vi "Edit_Batch.vi"(6 "error in (no error) 5":errorcluster, 7 "Batch Data 3":T1, 8 "Primery key names":string[](array[string]), 9 "Module Number  3":dbl=1.0, 10 "Batch data":string[](array[string]), 11 "Primery key last values":string[](array[string])) -> (0 "error out":errorcluster, 3 "Sucess ?":bool)   [LabVIEW 2015, in "Copy of Untitled Library 1.lvlib"]
uses:
  Copy of Untitled Library 1.lvlib
  Controls/Caller Queue Control .ctl
  Controls/Control 1.ctl
  Controls/Enum Constant.ctl
  <userlib>/origin_lib_main/db_interface/DB Operations Enum.ctl
  <userlib>/origin_lib_main/db_interface/DB Interface.lvlib
panel:
  in  "Cluster":T2
  out "concatenated string":string
  out "format string 2":string
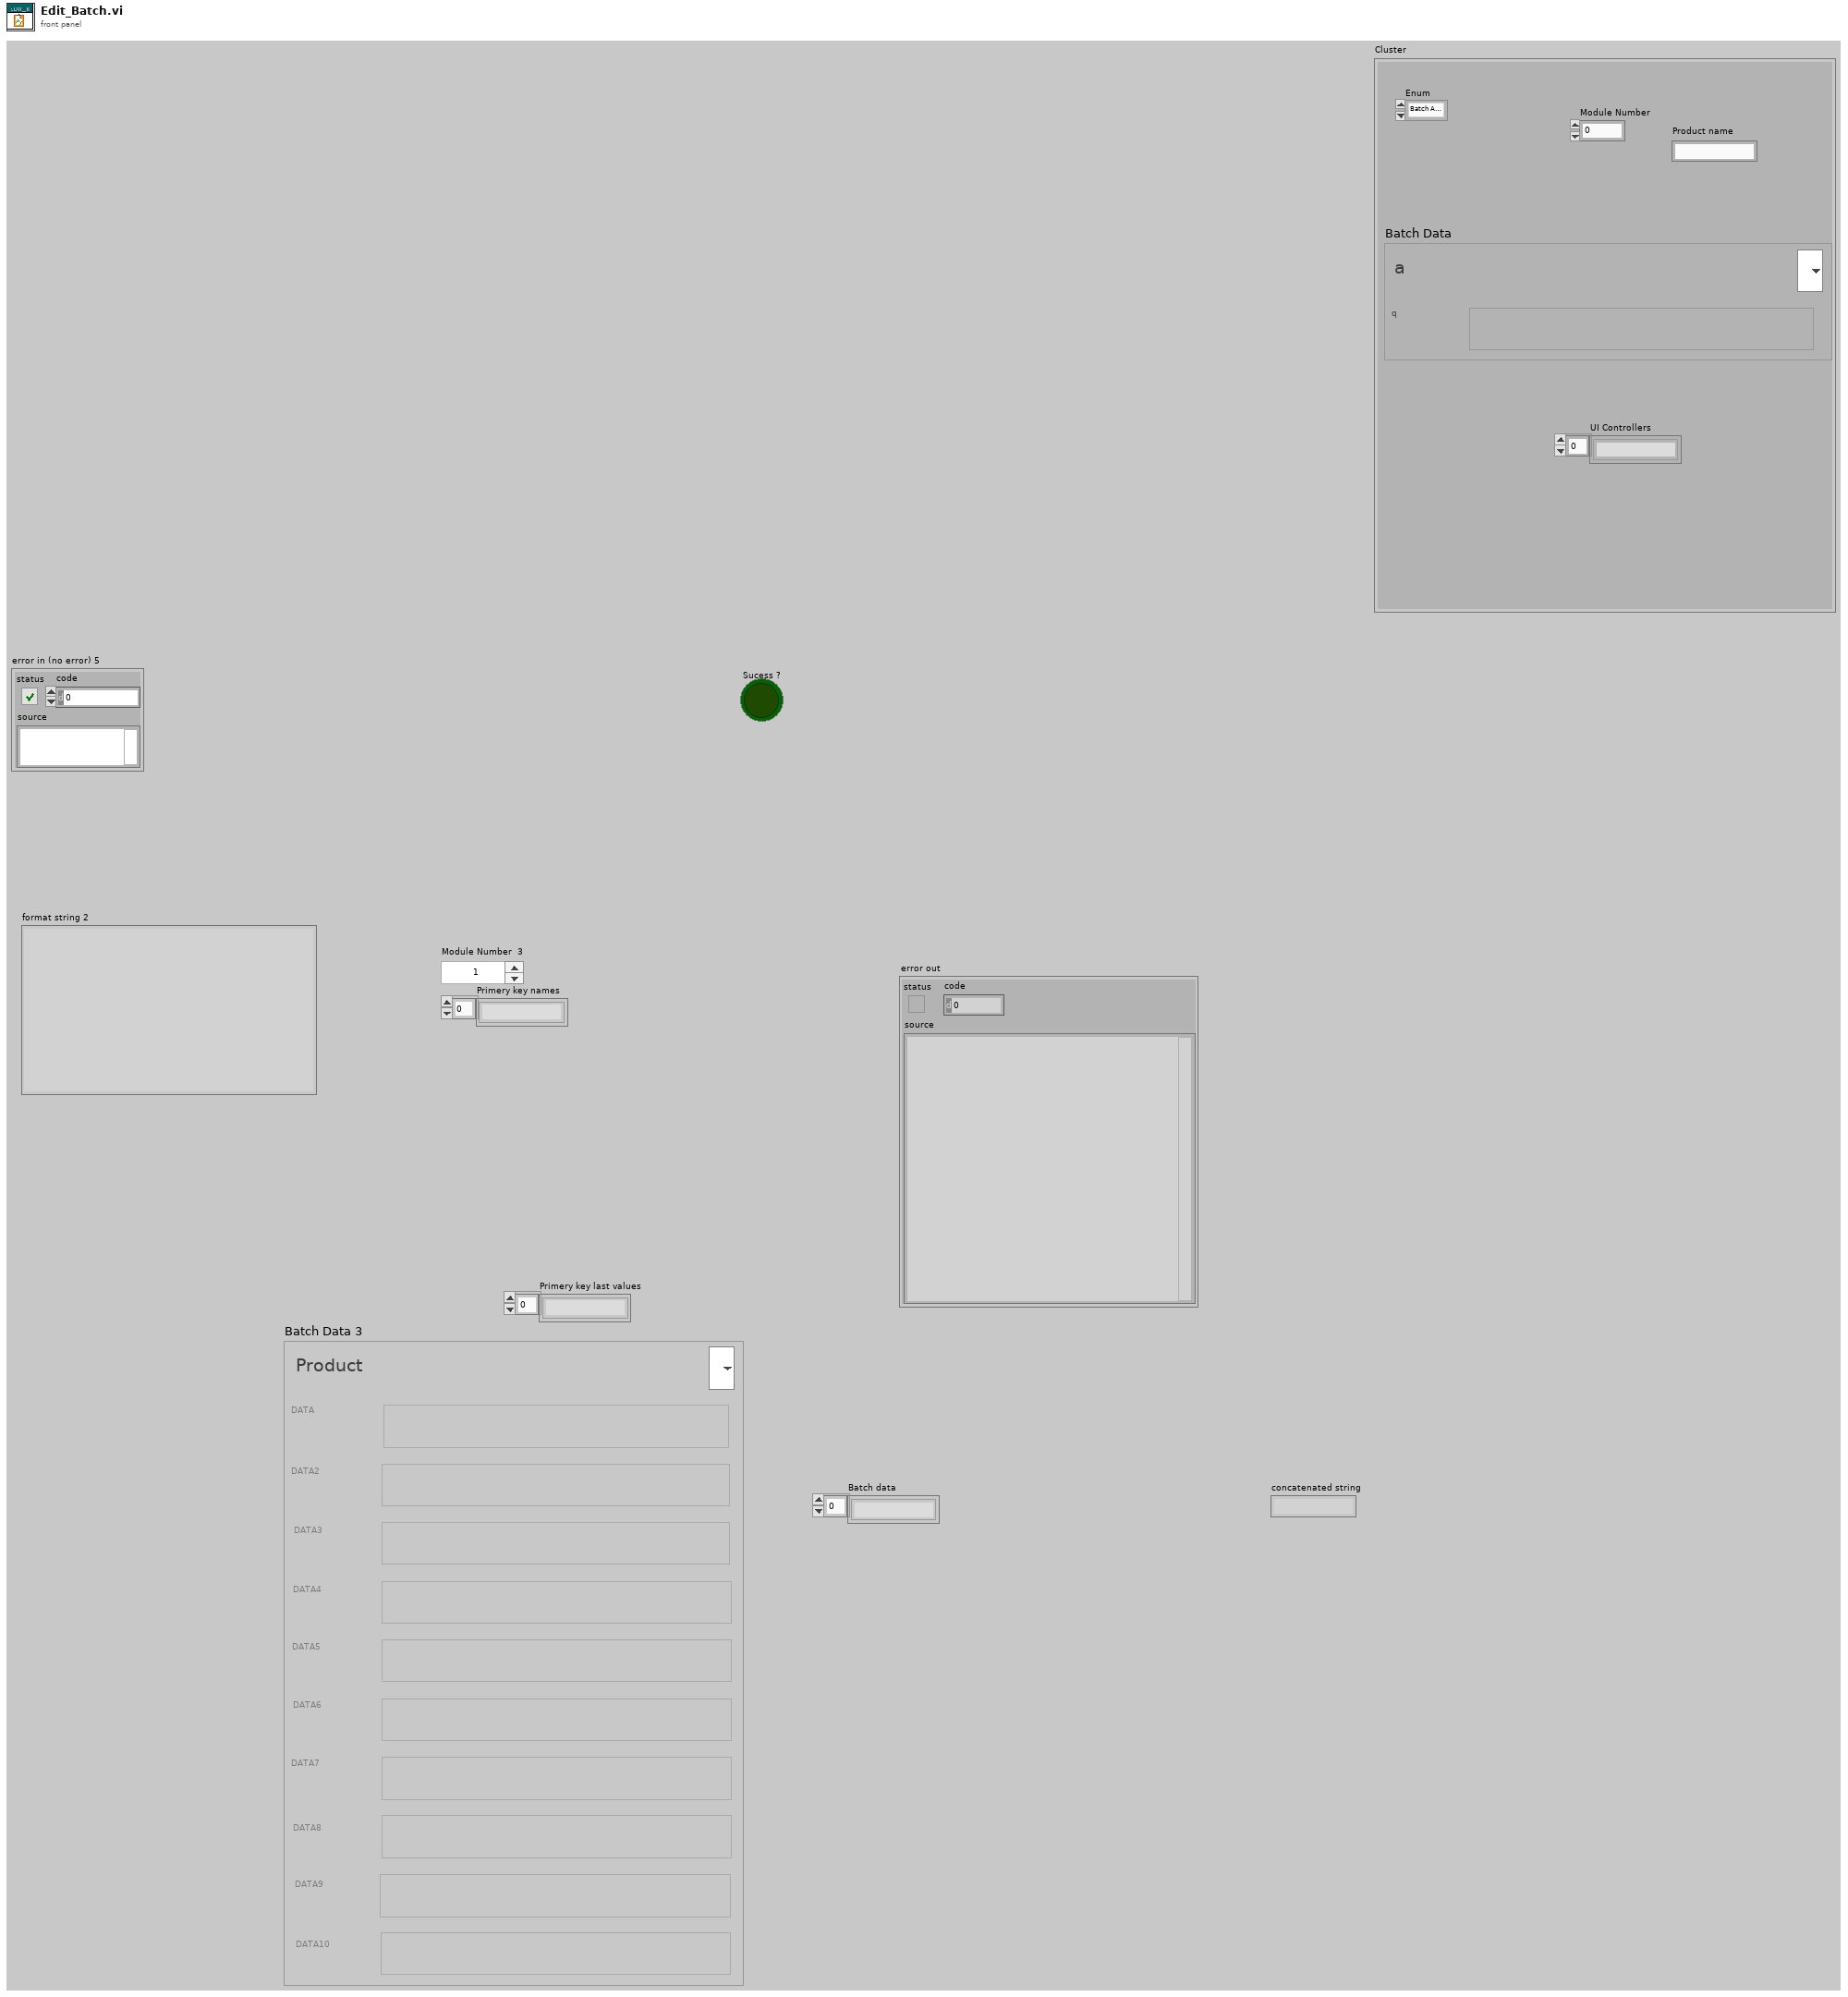
[diagram p1: front panel]
types:
  T1 = typedef "Copy of Untitled Library 1.lvlib/Control 1.ctl" = cluster{"DATA":string, "DATA 2":string, "DATA 3":string, "DATA 4":string, "DATA 5":string, "DATA 6":string, "DATA 7":string, "DATA 8":string, "DATA 9":string, "DATA 10":string, "Product":string}
  T2 = typedef "Caller Queue Control .ctl" = cluster{"Enum":enum16{"Batch Added", "Batch Deleted", "Batch Opened", "Batch Closed", "Batch Edited", "new Product Added", "Product deleted "}, "Batch Data 3":T1, "UI Controllers":string[], "Product name":string, "Module Number":dbl}
  T3 = typedef "DB Interface.lvlib/DB Operations Enum.ctl" = enum16{"Select", "Update", "Insert", "Delete", "Fetch SQL Query", "Execute SQL Query", "Drop Table", "List Tables"}
  T4 = typedef "Enum Constant.ctl" = enum16{"Init", "Read", "Write"}
  T5 = typedef "FGV Data.ctl" = T6[]
  T6 = typedef "FGV Cluster Data.ctl" = cluster{"Manual/Automatic":bool, "UI Controllers ":string[], "UI Primery Key ":dbl[], "Caller Queue & MSG":T7, "Module ID":dbl, "DB Reference In":T8, "Products Columns":string[], "Cluster":cluster{"Delete Product":enum8{"Enabled", "Disabled", "Disabled and Grayed Out"}, "Add Product ":enum8{"Enabled", "Disabled", "Disabled and Grayed Out"}, "EDIT BATCH":enum8{"Enabled", "Disabled", "Disabled and Grayed Out"}, "Open Batch ":enum8{"Enabled", "Disabled", "Disabled and Grayed Out"}, "Close Batch":enum8{"Enabled", "Disabled", "Disabled and Grayed Out"}, "Delete Batch":enum8{"Enabled", "Disabled", "Disabled and Grayed Out"}, "Add Batch ":enum8{"Enabled", "Disabled", "Disabled and Grayed Out"}}}
  T7 = typedef "Queue and Caller MSG.ctl" = cluster{"Caller Queue":refnum<queue>, "Caller MSG":string}
  T8 = typedef "NI_Database_API.lvlib/Conn ObjectReference.ctl" = refnum<k1>
  T9 = enum16{"Batch Added", "Batch Deleted", "Batch Opened", "Batch Closed", "Batch Edited", "new Product Added", "Product deleted "}
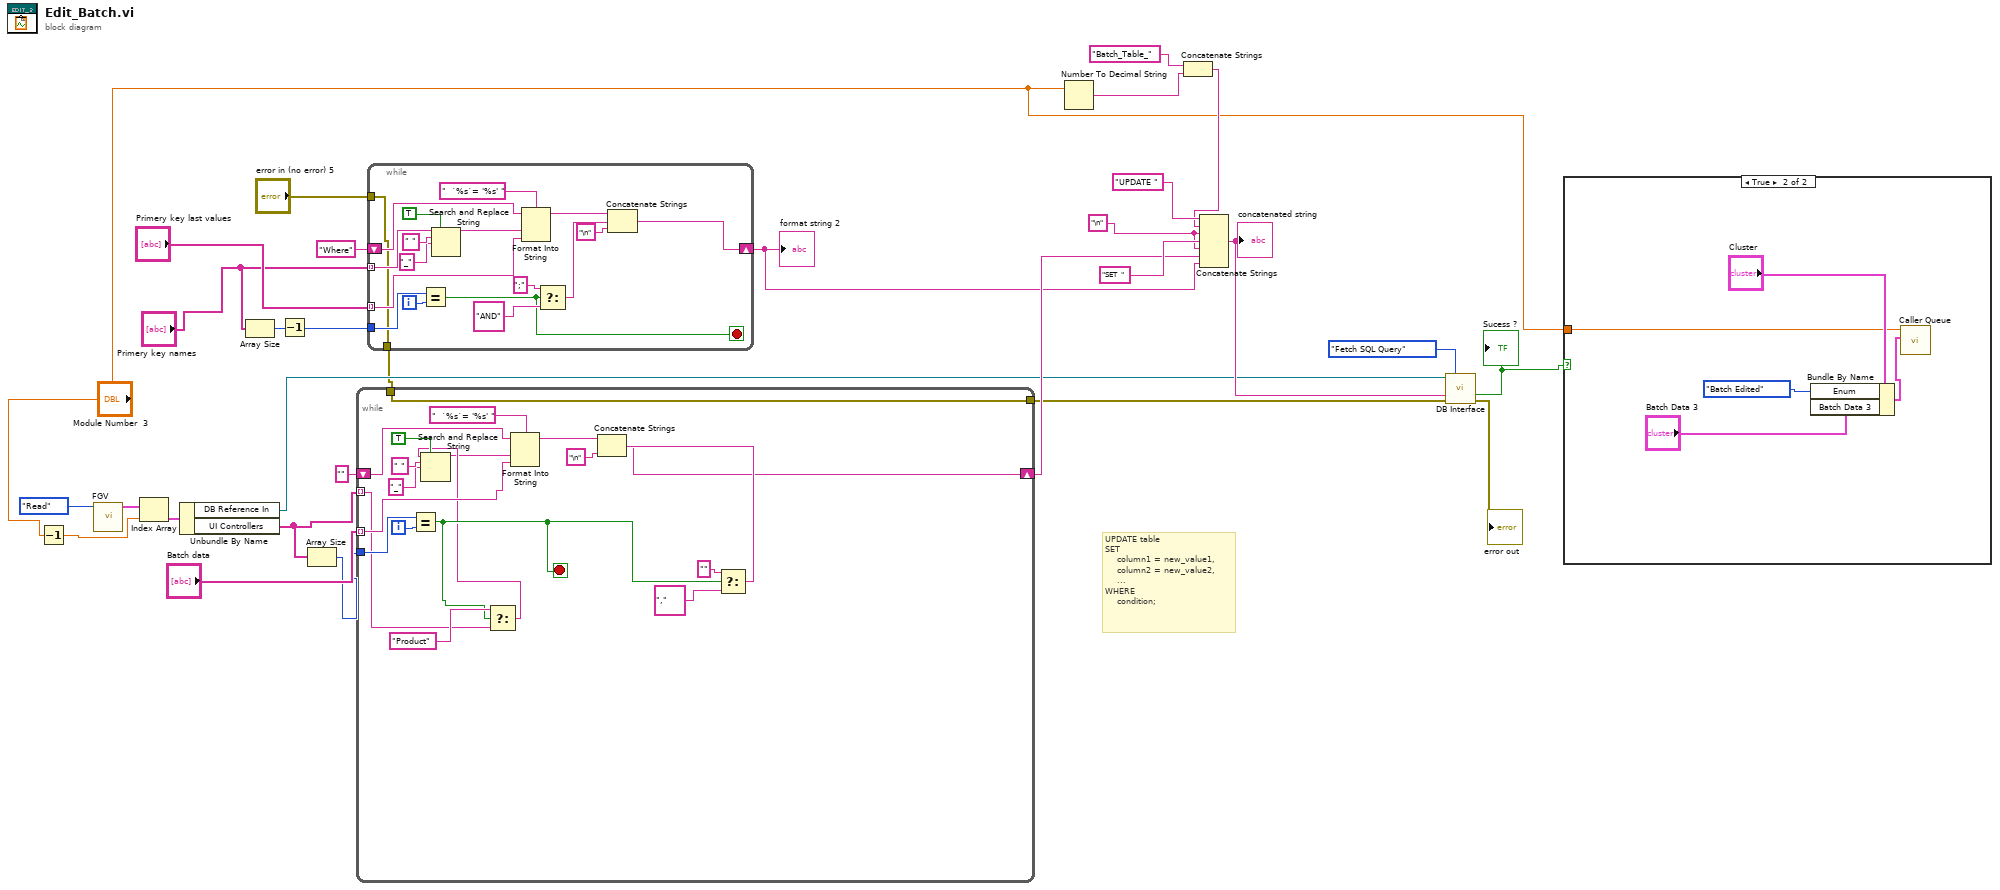
[diagram p0: block diagram]
diagram:
  w11 = "\n" ("string")
  # "UPDATE table\nSET \n    column1 = new_value1,\n    column2 = new_value2,\n    ...\nWHERE\n    condition;"
  n1 = Decrement(x="Module Number  3") -> (x-1=w19:dbl)
  n2 = call "FGV.vi"("Enum"=Enum_Constant."Read") -> ("Read Data"=w24:T5)  [unwired: 9 in, 1 out]
  n3 = Index Array(array=w24, index=w19) -> (element=w25:T6)
  n4 = Unbundle By Name(w25) -> ("DB Reference In"=w12:T8, "UI Controllers"=w8:string[])
  n5 = Array Size(array="Primery key names") -> (size(s)=w29:i32)
  n6 = Decrement(x=w29) -> (x-1=w28:i32)
  n7 = Array Size(array=w8) -> (size(s)=w3:i32)
  n8 = while {
    shift-right: [w35] -> w20
    shift-left: "Where" ("format string") -> [w47]
    tunnel: w28 -> [w41]
    tunnel: "Primery key names" -> [w36] mode=indexing
    tunnel: "Primery key last values" -> [w33] mode=indexing
    tunnel: [w31] -> w6
    tunnel: "error in (no error) 5" -> [w31]
    i -> [w42]
    stop <- w32 stop-if-true
    n9 = Equal?(x=w41, y=w42) -> (x = y?=w32:bool)
    n10 = Search and Replace String(replace all?=TRUE ("replace all? (F)"), input string=w36, search string=" ", replace string="_" ("replace string (\"\")")) -> (result string=w37:string)  [unwired: 4 in, 3 out]
    n11 = Format Into String(format string="  `%s`= '%s' ", initial string=w47, w37, w33) -> (resulting string=w46:string)  [unwired: 1 in, 1 out]
    n12 = Select(t=";", s=w32, f="AND") -> (s? t:f=w43:string)
    n13 = Concatenate Strings(w46, w43, "\n" ("string")) -> (w35:string)
  }
  "format string 2" <- w20
  n14 = while {
    shift-right: [w57] -> w21
    shift-left: "" -> [w67]
    tunnel: w3 -> [w61]
    tunnel: w8 -> [w51] mode=indexing
    tunnel: "Batch data" -> [w53] mode=indexing
    tunnel: w6 -> [w52]
    tunnel: [w52] -> w5
    i -> [w62]
    stop <- w54 stop-if-true
    n15 = Equal?(x=w61, y=w62) -> (x = y?=w54:bool)
    n16 = Select(t="Product", s=w54, f=w51) -> (s? t:f=w50:string)
    n17 = Search and Replace String(replace all?=TRUE ("replace all? (F)"), input string=w50, search string=" ", replace string="_" ("replace string (\"\")")) -> (result string=w49:string)  [unwired: 4 in, 3 out]
    n18 = Format Into String(format string="  `%s`= '%s' ", initial string=w67, w49, w53) -> (resulting string=w66:string)  [unwired: 1 in, 1 out]
    n19 = Select(t="", s=w54, f=",") -> (s? t:f=w63:string)
    n20 = Concatenate Strings(w66, w63, "\n" ("string")) -> (w57:string)
  }
  n21 = Number To Decimal String(number="Module Number  3") -> (decimal integer string=w17:string)  [unwired: 1 in]
  n22 = Concatenate Strings("Batch_Table_" ("string"), w17) -> (w16:string)
  n23 = Concatenate Strings("UPDATE " ("string"), w16, w11, "SET  " ("string"), w11, w21, w20) -> (w14:string)
  "concatenated string" <- w14
  n24 = call <userlib>:"DB Interface.vi"("DB Ref In"=w12, "Operation"=DB_Operations_Enum."Fetch SQL Query", "SQL Query"=w14, "error in (no error)"=w5) -> ("Sucess ?"=w1:bool, "error out"=→"error out":errorcluster)  [unwired: 8 in, 2 out]
  "Sucess ?" <- w1
  n25 = case shown="True" w1 {
    tunnel: "Module Number  3" -> [_ w71]
    frame False {
    }
    frame True {
      n26 = Bundle By Name(cluster="Cluster", "Enum"=T9."Batch Edited", "Batch Data 3"="Batch Data 3") -> (w69:T2)
      n27 = call "Caller Queue .vi"("Cluster"=w69, "Module Number  3"=w71) -> ()  [unwired: 9 in, 1 out]
    }
  }
